vi "Echo_Autonomous_Independent.vi"() -> (5 "End of file":bool, 7 "Output 10":dbl, 9 "Output 9":dbl, 11 "Output 8":dbl, 13 "Output 7":dbl, 14 "Output 1":dbl, 15 "Output 2":dbl, 16 "Output 3":dbl, 17 "Output 4":dbl, 18 "Output 5":dbl, 19 "Output 6":dbl)   [LabVIEW 2012]
uses:
  Echo_Global_Data.vi
panel:
  # "Outputs somewhere in autonomous independent"
  # "This VI takes reads into an array,\nEcho Combined Data, and sets\nthe outputs to the correct values"
  # "Has the last file been\ncompletely read?"
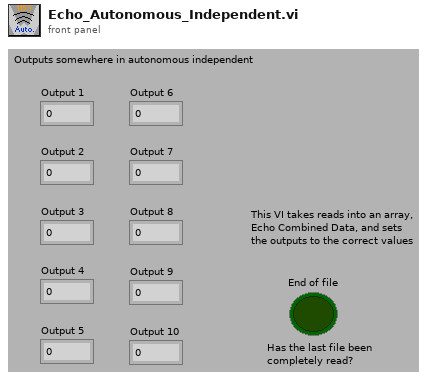
[diagram p1: front panel]
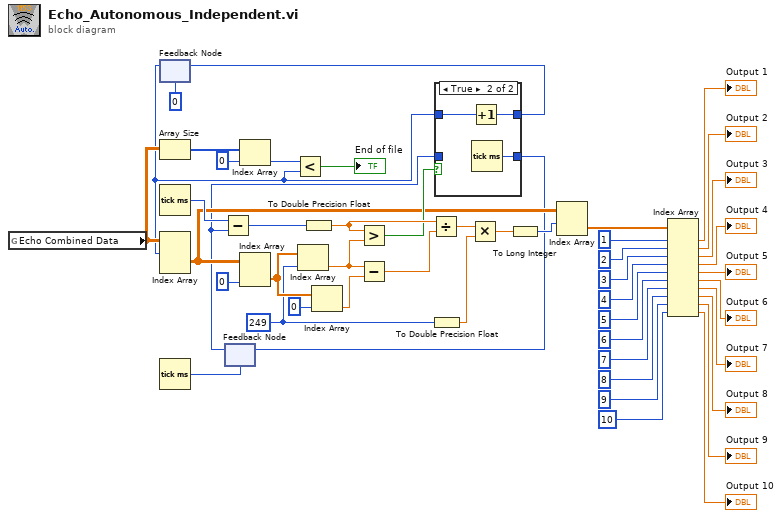
[diagram p0: block diagram]
diagram:
  w41 = 249 ("number")
  n1 = global read "Echo_Global_Data.vi" "Echo Combined Data"() -> (w6:dbl[][][])
  n2 = feedback #1(0) -> (w1:i32)
  n3 = Array Size(array=w6) -> (size(s)=w5:i32[])
  n4 = Tick Count (ms)() -> (millisecond timer value=w40:u32)
  n5 = Index Array(array=w6, index (dim 0)=w1) -> (element=w22:dbl[][])  [unwired: 2 in]
  n6 = Tick Count (ms)() -> (millisecond timer value=w18:u32)
  n7 = feedback #2(w18) -> (w17:u32)
  n8 = Subtract(x=w40, y=w17) -> (x-y=w39:u32)
  n9 = Index Array(array=w5, index=0) -> (element=w3:i32)
  n10 = Index Array(array=w22, index (col)=0) -> (element=w47:dbl[])  [unwired: 1 in]
  n11 = Less?(x=w3, y=w1) -> (x < y?=→"End of file":bool)
  n12 = Index Array(array=w47, index=w41) -> (element=w44:dbl)
  n13 = To Double Precision Float(number=w39) -> (double precision float=w38:dbl)
  n14 = Index Array(array=w47, index=0) -> (element=w46:dbl)
  n15 = Greater?(x=w38, y=w44) -> (0:w23:bool)
  n16 = Subtract(x=w44, y=w46) -> (x-y=w45:dbl)
  n17 = Divide(x=w38, y=w45) -> (x/y=w37:dbl)
  n18 = To Double Precision Float(number=w41) -> (double precision float=w43:dbl)
  n19 = case shown="True" w23 {
    tunnel: w1 -> [w50 w53]
    tunnel: [w50 w52] -> w21
    tunnel: [w49 w51] -> w19
    tunnel: w17 -> [w49 _]
    frame False {
    }
    frame True {
      n20 = Increment(x=w53) -> (x+1=w52:i32)
      n21 = Tick Count (ms)() -> (millisecond timer value=w51:u32)
    }
  }
  n22 = feedback-in #1(w21) -> ()
  n23 = feedback-in #2(w19) -> ()
  n24 = Multiply(x=w37, y=w43) -> (x*y=w36:dbl)
  n25 = To Long Integer(number=w36) -> (32bit integer=w35:i32)
  n26 = Index Array(array=w22, index (row)=w35) -> (element=w33:dbl[])  [unwired: 1 in]
  n27 = Index Array(array=w33, index #1=1, index #2=2, index #3=3, index #4=4, index #5=5, index #6=6, index #7=7, index #8=8, index #9=9, index #10=10) -> (element #1=→"Output 1":dbl, element #2=→"Output 2":dbl, element #3=→"Output 3":dbl, element #4=→"Output 4":dbl, element #5=→"Output 5":dbl, element #6=→"Output 6":dbl, element #7=→"Output 7":dbl, element #8=→"Output 8":dbl, element #9=→"Output 9":dbl, element #10=→"Output 10":dbl)
